vi "Assert Collection Not Empty.vi"(7 "Message (\"\")":string, 8 "error in (no error)":errorcluster, 10 "Collection":variant) -> (0 "error out":errorcluster)   [LabVIEW 2017, in "Transparent Assertions.lvlib" / "Assertions.lvlib"]
doc: "Asserts that a collection (array, set, or map) is not empty. Returns an error if the assertion fails, and optionally appends a custom message to the error."
uses:
  Assertions.lvlib
  Constraints/Collection Is Empty/Collection Is Empty.lvclass
  C:/Users/pasca/Projects/Home/TransparentAssertions/src/Transparent Assertions/Constraints/Constraint/Constraint.lvclass
  Constraints/LogicalNot/LogicalNot.lvclass
  Constraints/UnaryOperator/UnaryOperator.lvclass
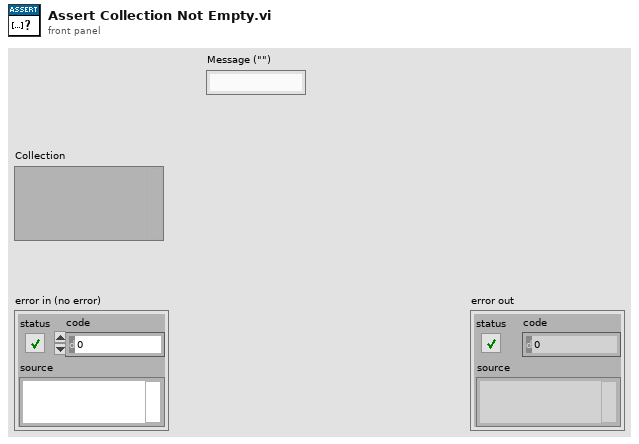
[diagram p1: front panel]
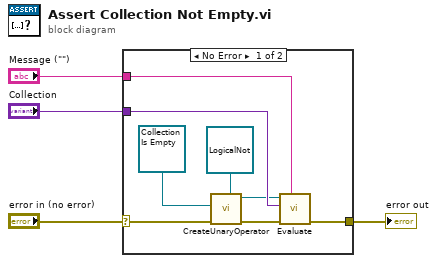
[diagram p0: block diagram]
diagram:
  n1 = case shown="No Error" "error in (no error)" {
    selector: "error in (no error)" -> [w9 w13]
    tunnel: [w12 w13] -> w4
    tunnel: "Collection" -> [w11 _]
    tunnel: "Message (\"\")" -> [w10 _]
    frame No Error {
      n2 = call-dynamic "CreateUnaryOperator.vi"("UnaryOperator In"=refnum<class "LogicalNot.lvclass"> refnum ("Transparent Assertions.lvlib:Constraints.lvlib:LogicalNot.lvclass"), "error in (no error)"=w9, "Constraint"=refnum<class "Collection Is Empty.lvclass"> refnum ("Transparent Assertions.lvlib:Constraints.lvlib:Collection Is Empty.lvclass")) -> ("error out"=w8:errorcluster, "UnaryOperator"=w6:refnum<class "UnaryOperator.lvclass">)  [unwired: 7 in]
      n3 = call-dynamic "Evaluate.vi"("Message (\"\")"=w10, "error in (no error)"=w8, "Actual"=w11, "Constraint in"=w6) -> ("error out"=w12:errorcluster)  [unwired: 6 in, 1 out]
    }
    frame Error {
    }
  }
  "error out" <- w4
